vi "Picture Zoom.vi"(0 "Picture in":refnum<vi>, 1 "image data":T1, 5 "error in":errorcluster) -> (19 "error out":errorcluster)   [LabVIEW 2024]
uses:
  <vilib>/picture/picture.llb/imagedata.ctl
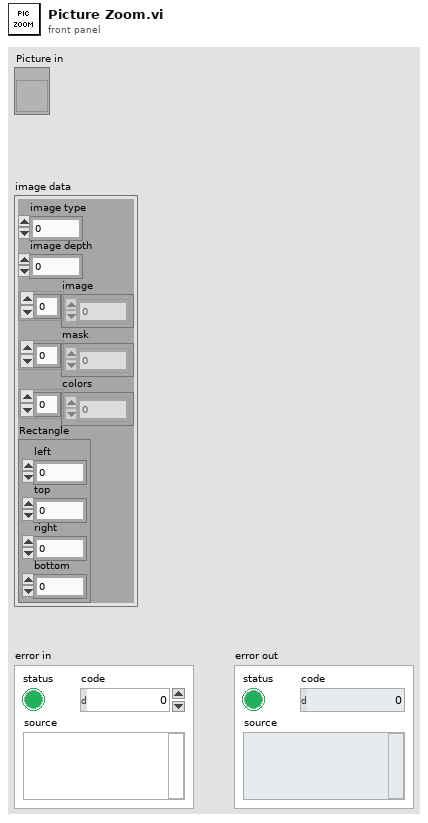
[diagram p1: front panel]
types:
  T1 = typedef "imagedata.ctl" = cluster{"image type":i32, "image depth":i32, "image":u8[], "mask":u8[], "colors":u32[], "Rectangle":cluster{"left":i16, "top":i16, "right":i16, "bottom":i16}}
  T2 = typedef "LVBoundsTypeDef.ctl" = cluster{"Width":u32, "Height":u32}
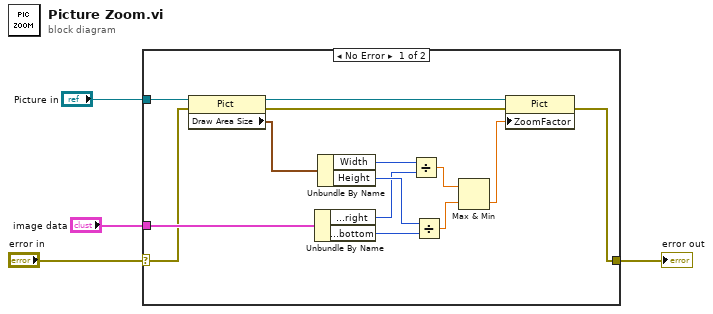
[diagram p0: block diagram]
diagram:
  n1 = case shown="No Error" "error in" {
    selector: "error in" -> [w6 w19]
    tunnel: "image data" -> [w18 _]
    tunnel: "Picture in" -> [w9 _]
    tunnel: [w5 w19] -> w1
    frame No Error {
      n2 = property on="Property Node" class="Pict"(reference=w9, error in=w6) -> (reference out=w8:refnum<vi>, error out=w7:errorcluster, "Draw Area Size"=w14:T2)
      n3 = Unbundle By Name(w18) -> ("Rectangle.right"=w10:i16, "Rectangle.bottom"=w11:i16)
      n4 = Unbundle By Name(w14) -> ("Width"=w15:u32, "Height"=w16:u32)
      n5 = Divide(x=w15, y=w10) -> (x/y=w13:dbl)
      n6 = Divide(x=w16, y=w11) -> (x/y=w12:dbl)
      n7 = Max & Min(x=w13, y=w12) -> (min(x,y)=w17:dbl)  [unwired: 1 out]
      n8 = property on="Property Node" class="Pict"(reference=w8, error in=w7, "ZoomFactor"=w17) -> (error out=w5:errorcluster)  [unwired: 1 out]
    }
    frame Error {
    }
  }
  "error out" <- w1
